vi "Stop Core.vi"(10 "final error code":i32, 11 "TEC Controller in":refnum<class "TEC Controller.lvclass">) -> (3 "TEC Controller out":refnum<class "TEC Controller.lvclass">)   [LabVIEW 2014, in "Humidifier Test Lib.lvlib" / "TEC Controller.lvclass"]
doc: "(<B>Filename</B>: Actor Framework.lvlib:Actor.lvclass:Stop Core.vi)\n\nDefines what the actor does before it stops. Use the <B>final error code</B> input to determine whether the actor shut down in response to an error.\n\nBy default, this method does nothing. A descendant class may override it to define behavior, such as shutting down any processes the actor initiated in its override of the Actor Core method."
uses:
  TEC Controller.lvclass
  reusable/Session APIs/File Access/Config Data/Config Data.lvclass
  TEC Controller.lvclass/TEC Controller.ctl
  <vilib>/ActorFramework/Actor/Actor.lvclass
  <userlib>/_Session Fwk/Session - Root.lvclass
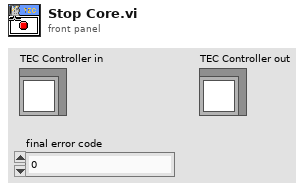
[diagram p1: front panel]
types:
  T1 = typedef "Session - Root.lvclass/Session Handle.ctl" = refnum<data-value>
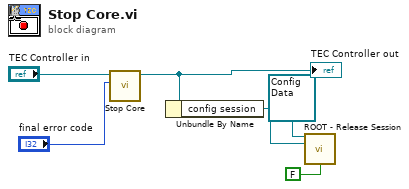
[diagram p0: block diagram]
diagram:
  n1 = call-parent "Stop Core.vi"("final error code"="final error code", "Actor in"="TEC Controller in") -> ("Actor out"=w4:refnum<class "TEC Controller.lvclass">)  [unwired: 9 in]
  "TEC Controller out" <- w4
  n2 = Unbundle By Name(w4) -> ("config session"=w3:T1)
  n3 = call <userlib>:"ROOT - Release Session.vi"("OBJ - Session in"=refnum<class "Config Data.lvclass"> refnum ("Config Data"), "Session Handle in"=w3, "force destroy? (F)"=FALSE) -> ()  [unwired: 11 in, 2 out]
